vi "Actor Core.vi"(8 "error in":errorcluster, 11 "Gage digitizer actor in":refnum<class "Gage digitizer actor.lvclass">) -> (0 "error out":errorcluster, 3 "Actor out":refnum<class "Actor.lvclass">)   [LabVIEW 2015, in "Gage digitizer actor.lvclass"]
doc: "(<B>Filename</B>: Actor Framework.lvlib:Actor.lvclass:Actor Core.vi)\n\nReceives messages to the actor, reacts to them, and initiates any error handling that may shut the actor down.\n\nDescendant classes may override this VI to append parallel tasks for the actor to complete while it handles messages. Overrides use the Call Parent Method node."
uses:
  Gage digitizer actor.lvclass
  <vilib>/ActorFramework/Actor/Actor.lvclass
  Gage digitizer actor.lvclass/Gage digitizer actor.ctl
  Measure_core/Measure Object/Measure Object.lvclass/Measure Object.ctl
  Measure_core/Measure Object/Read stop event.vi
  Measure_core/Pulse Recorders/Pulse Recorder/Pulse Recorder.lvclass
panel:
  in  "Live monitor":bool
  out "Waveform Graph":waveform(dbl)(graph)
  in  "Configuration":T1={"Number of points"=816000.0, "Input Range"=10000, "Trigger Level"=29, "Trigger source"=TRUE} {"Trigger Level" min=-100 max=100 step=1 scale=-100.0..100.0; "Input Range" items=["+/- 5 V"=10000, "+/- 2 V"=4000, "+/- 1 V"=2000, "+/- 500 mV"=1000, "+/- 200 mV"=400, "+/- 100 mV"=200]; "Number of points" min=160.0 step=160.0}
  # "Basic Card Controlls"
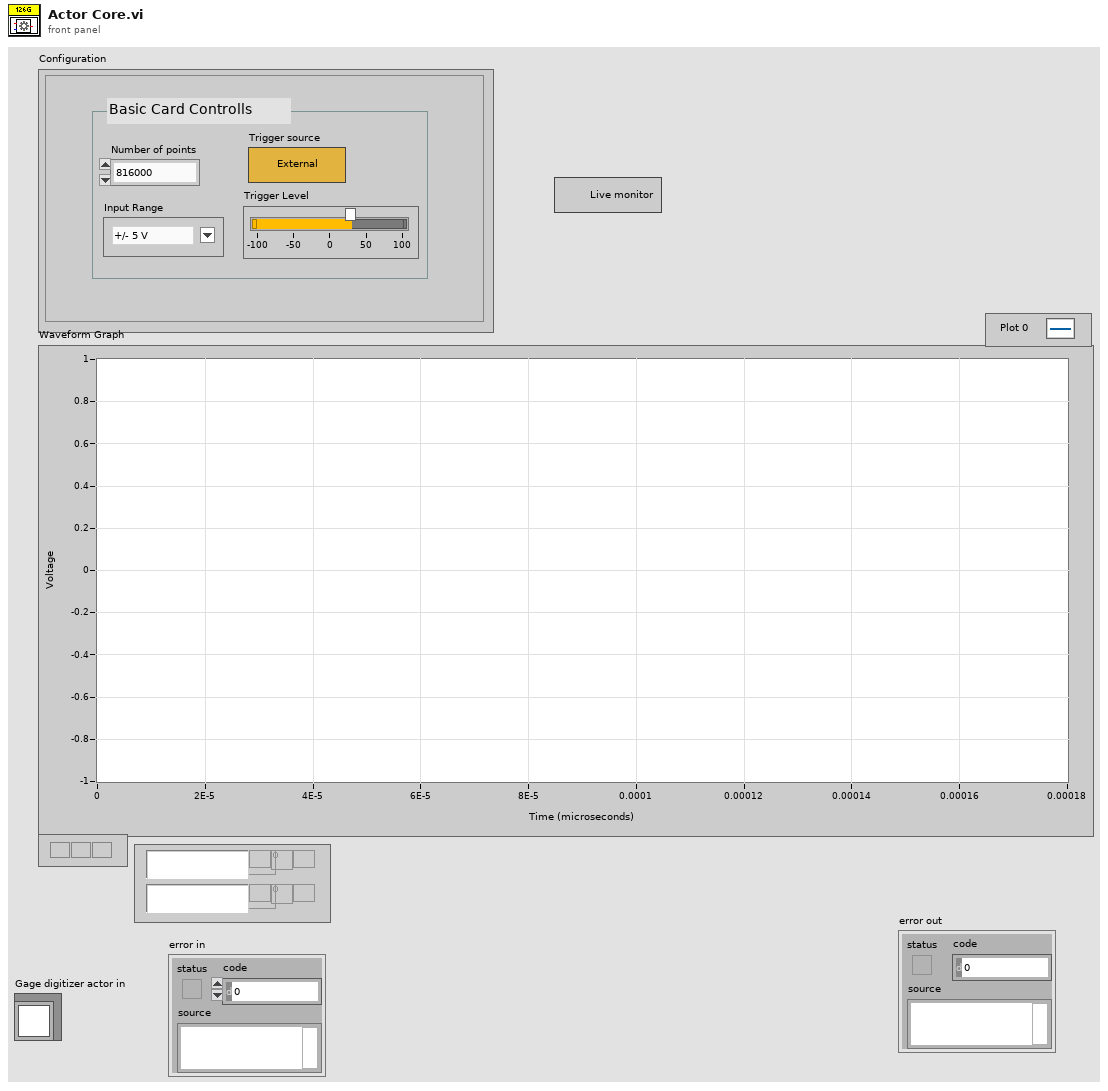
[diagram p1: front panel]
types:
  T1 = cluster{"Number of points":dbl, "Input Range":u32, "Trigger Level":i32, "Trigger source":bool}
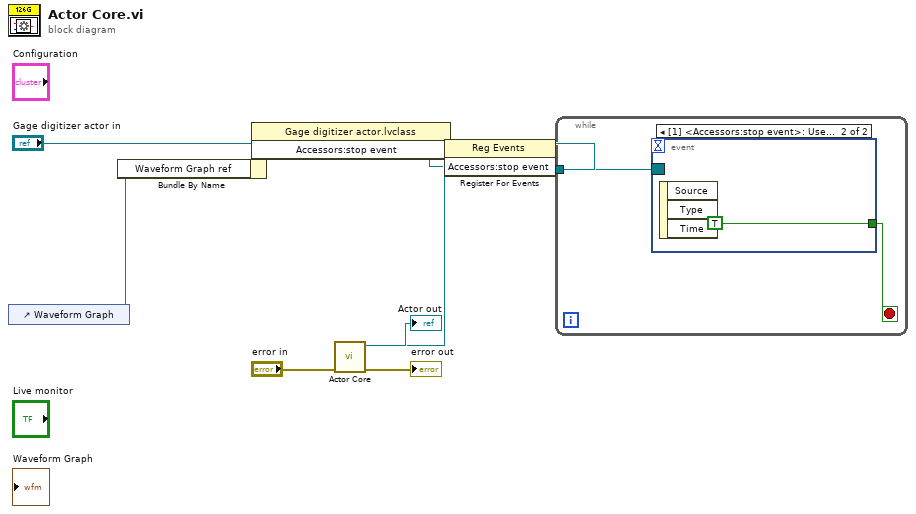
[diagram p0: block diagram]
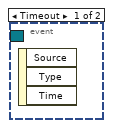
[diagram p2: hidden frame]
diagram:
  n1 = control-ref of="Waveform Graph"() -> (w4:refnum<vi>)
  n2 = Bundle By Name(cluster="Gage digitizer actor in", "Waveform Graph ref"=w4) -> (w5:refnum<class "Gage digitizer actor.lvclass">)
  n3 = property class="Gage digitizer actor.lvclass"(reference=w5) -> (reference out=w3:refnum<class "Gage digitizer actor.lvclass">, "Accessors:stop event"=w2:refnum<user-event>)  [unwired: 1 in, 1 out]
  n4 = call-parent "Actor Core.vi"("error in"="error in", "Pulse Recorder in"=w3) -> ("error out"=→"error out":errorcluster, "Actor out"=→"Actor out":refnum<class "Actor.lvclass">)  [unwired: 8 in]
  n5 = register-events(w2) -> (reference out=w1:refnum<event-registration>)  [unwired: 2 in, 1 out]
  n6 = while {
    tunnel: w1 -> [w11]
    stop <- w10 stop-if-true
    n7 = event shown="[1] <Accessors:stop event>: User Event" {
      selector: w11 -> [_ _]
      dyn-events: _ -> [_ _]
      timeout: _ -> [_ _]
      tunnel: [_ TRUE] -> w10
      event Timeout {
        n8 = event-data() -> ()  [unwired: 1 in, 3 out]
      }
      event User Event {
        n9 = event-data() -> ()  [unwired: 1 in, 3 out]
      }
    }
  }
